vi "parse_point_cloud.vi"(4 "error in":errorcluster, 7 "msg in":string) -> (0 "error out":errorcluster, 1 "Header":T1, 2 "Point Cloud":T2, 3 "msg out":string)   [LabVIEW 2010]
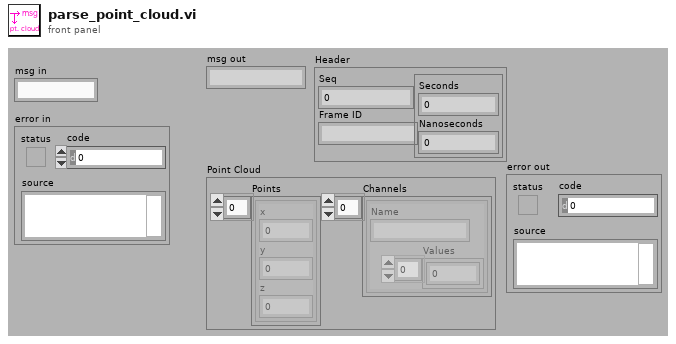
[diagram p1: front panel]
types:
  T1 = cluster{"Seq":u32, "Frame ID":string, cluster{"Seconds":i32, "Nanoseconds":i32}}
  T2 = cluster{"Points":cluster{"x":sgl, "y":sgl, "z":sgl}[], "Channels":cluster{"Name":string, "Values":sgl[]}[]}
  T3 = cluster{"Seq":u32, "Frame ID":string, "Timestamp":cluster{"Seconds":i32, "Nanoseconds":i32}}
  T4 = cluster{cluster{"x":sgl, "y":sgl, "z":sgl}[], cluster{"Name":string, "Values":sgl[]}[]}
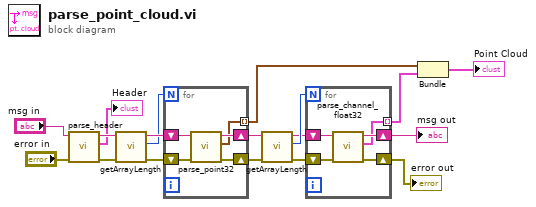
[diagram p0: block diagram]
diagram:
  n1 = call "parse_header.vi"("error in"="error in", "msg in"="msg in") -> ("error out"=w5:errorcluster, "Header"=→"Header":T3, "msg out"=w17:string)  [unwired: 3 in]
  n2 = call "getArrayLength.vi"("error in"=w5, "msg in"=w17) -> ("error out"=w6:errorcluster, "array length"=w15:u32, "msg out"=w16:string)  [unwired: 3 in]
  n3 = for {
    N: w15 -> [_]
    shift-right: [w22] -> w14
    shift-left: w16 -> [w23]
    tunnel: [w21] -> w9 mode=indexing
    shift-right: [w19] -> w4
    shift-left: w6 -> [w20]
    n4 = call "parse_point32.vi"("error in"=w20, "msg in"=w23) -> ("error out"=w19:errorcluster, "Point32"=w21:cluster{"x":sgl, "y":sgl, "z":sgl}, "msg out"=w22:string)  [unwired: 3 in]
  }
  n5 = call "getArrayLength.vi"("error in"=w4, "msg in"=w14) -> ("error out"=w3:errorcluster, "array length"=w13:u32, "msg out"=w12:string)  [unwired: 3 in]
  n6 = for {
    N: w13 -> [_]
    shift-right: [w27] -> w11
    shift-left: w12 -> [w28]
    tunnel: [w26] -> w10 mode=indexing
    shift-right: [w24] -> w2
    shift-left: w3 -> [w25]
    n7 = call "parse_channel_float32.vi"("error in"=w25, "msg in"=w28) -> ("error out"=w24:errorcluster, "ChannelFloat32"=w26:cluster{"Name":string, "Values":sgl[]}, "msg out"=w27:string)  [unwired: 3 in]
  }
  "msg out" <- w11
  "error out" <- w2
  n8 = Bundle(w9, w10) -> (→"Point Cloud":T4)  [unwired: 1 in]
